vi "FormatDoubleToString.vi"(0 "Double":dbl, 1 "Precision (3)":i16=3) -> (15 "String":string)   [LabVIEW 2014]
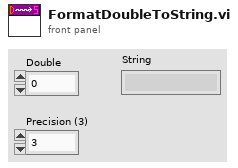
[diagram p1: front panel]
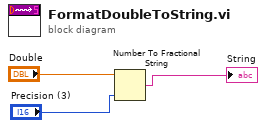
[diagram p0: block diagram]
diagram:
  n1 = Number To Fractional String(number="Double", precision (6)="Precision (3)") -> (F-format string=→"String":string)  [unwired: 2 in]
